vi "Set Minimum Log Level.vi"(10 "minimum log level":T1, 11 "logger in":refnum<class "Logger.lvclass">) -> (3 "logger out":refnum<class "Logger.lvclass">)   [LabVIEW 2018, in "GLog.lvlib" / "Logger.lvclass"]
uses:
  Logger.lvclass
  Log Levels.ctl
  Logger.lvclass/Logger.ctl
panel:
  # "Connector Pane"
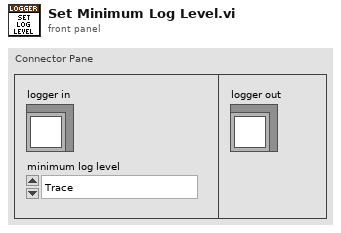
[diagram p1: front panel]
types:
  T1 = typedef "GLog.lvlib/Logger.lvclass/Log Levels.ctl" = enum16{"Trace", "Debug", "Info", "Warning", "Error", "Critical"}
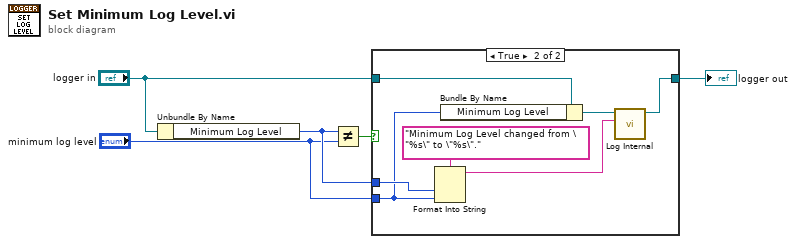
[diagram p0: block diagram]
diagram:
  n1 = Unbundle By Name("logger in") -> ("Minimum Log Level"=w2:T1)
  n2 = Not Equal?(x=w2, y="minimum log level") -> (x != y?=w3:bool)
  n3 = case shown="True" w3 {
    tunnel: [w6 w12] -> w5
    tunnel: "logger in" -> [w6 w10]
    tunnel: w2 -> [_ w9]
    tunnel: "minimum log level" -> [_ w7]
    frame False {
    }
    frame True {
      n4 = Format Into String(format string="Minimum Log Level changed from \"%s\" to \"%s\".", w9, w7) -> (resulting string=w8:string)  [unwired: 2 in, 1 out]
      n5 = Bundle By Name(cluster=w10, "Minimum Log Level"=w7) -> (w13:refnum<class "Logger.lvclass">)
      n6 = call "Log Internal.vi"("message"=w8, "logger in"=w13) -> ("logger out"=w12:refnum<class "Logger.lvclass">)  [unwired: 9 in]
    }
  }
  "logger out" <- w5
